vi "Drive Global.vi"() -> ()   [LabVIEW 2013]
panel:
  in  "Drive Info":T1
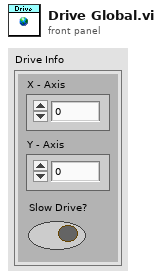
[diagram p1: front panel]
types:
  T1 = cluster{"X - Axis":dbl, "Y - Axis":dbl, "Slow Drive?":bool}
diagram:
